vi "Untitled 2.vi"() -> ()   [LabVIEW 2013]
uses:
  <vilib>/Rock Robotics/WPI/Joystick/WPI_JoystickGetSetRefNum.vi
panel:
  in  "Arm Position":enum16{"Arms open", "Arms closed"}(ring)
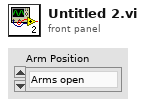
[diagram p1: front panel]
types:
  T1 = typedef "WPI_JoystickDevRef.ctl" = cluster{"Device":T2}
  T2 = typedef "WPI_JoystickDeviceEnum.ctl" = enum16{"USB 1", "USB 2", "USB 3", "USB 4", "Kinect 1", "Kinect 2"}
  T3 = typedef "WPI_JoystickButtonState.ctl" = cluster{"Button 1":bool, "Button 2":bool, "Button 3":bool, "Button 4":bool, "Button 5":bool, "Button 6":bool, "Button 7":bool, "Button 8":bool, "Button 9":bool, "Button 10":bool, "Button 11":bool, "Button 12":bool}
  T4 = typedef "WPI_DigitalInputDevRef.ctl" = cluster{"DevStatus":errorcluster, "DIO Channel":T5, "Digital Module":T6}
  T5 = typedef "FPGA_DIOChannel.ctl" = enum8{"DIO 1", "DIO 2", "DIO 3", "DIO 4", "DIO 5", "DIO 6", "DIO 7", "DIO 8", "DIO 9", "DIO 10", "DIO 11", "DIO 12", "DIO 13", "DIO 14", "Invalid"}
  T6 = typedef "FPGA_TypedefDigitalModule.ctl" = enum16{"Digital Module 1", "Digital Module 2"}
  T7 = typedef "WPI_MotorControlDeviceRef.ctl" = cluster{"DeviceStatus":errorcluster, "Type":enum16{"PWM", "CAN"}, "PWM":cluster{"Digital Module":T6, "PWM Channel":T8, "DeadBand":T9}, "CAN":cluster{"Device Number":u8, "Control Mode":T10, "Semaphore":T11, "Max Vout":dbl}, "Invert":bool, "TransformRef":T12, "InvTransformRef":T12}
  T8 = typedef "FPGA_DIOPWMChannel.ctl" = enum8{"PWM 1", "PWM 2", "PWM 3", "PWM 4", "PWM 5", "PWM 6", "PWM 7", "PWM 8", "PWM 9", "PWM 10", "Invalid"}
  T9 = typedef "WPI_PWMDeadband.ctl" = cluster{"Name":string, "maxPositivePwm":i32, "minPositivePwm":i32, "centerPwm":i32, "maxNegativePwm":i32, "minNegativePwm":i32, "angularRange":u16}
  T10 = typedef "WPI_CANJaguar_ControlMode.ctl" = enum8{"Percent VBus", "Current", "Speed", "Position", "Voltage"}
  T11 = typedef "Semaphore RefNum" = refnum<k1>
  T12 = typedef "WPI_PWMTransform_ConPane.ctl" = refnum<vi>
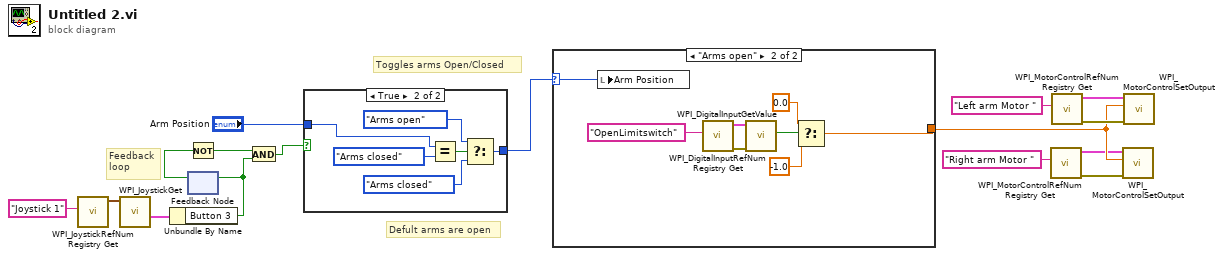
[diagram p0: block diagram]
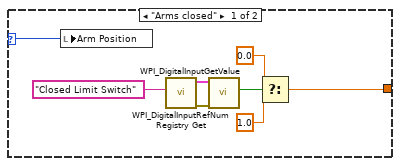
[diagram p3: hidden frame]
diagram:
  # "Toggles arms Open/Closed"
  # "Feedback\nloop"
  # "Defult arms are open"
  n1 = call <vilib>:"WPI_JoystickRefNum Registry Get.vi"("refnum name"="Joystick 1") -> ("JoystickDevRef"=w16:T1)  [unwired: 9 in, 1 out]
  n2 = call <vilib>:"WPI_JoystickGet.vi"("JoystickDevRef"=w16) -> ("Buttons"=w14:T3)  [unwired: 4 in, 2 out]
  n3 = Unbundle By Name(w14) -> ("Button 3"=w3:bool)
  n4 = feedback-in #1(w3) -> ()
  n5 = feedback #1() -> (w5:bool)  [unwired: 1 in]
  n6 = Not(x=w5) -> (.not. x?=w4:bool)
  n7 = And(x=w4, y=w3) -> (x .and. y?=w1:bool)
  n8 = case shown="True" w1 {
    tunnel: [w17 w23] -> w13
    tunnel: "Arm Position" -> [w17 w18]
    frame False {
    }
    frame True {
      n9 = Equal?(x=w18, y=enum16{"Arms open", "Arms closed"}."Arms closed") -> (x = y?=w21:bool)
      n10 = Select(t=enum16{"Arms open", "Arms closed"}."Arms open", s=w21, f=enum16{"Arms open", "Arms closed"}."Arms closed") -> (s? t:f=w23:enum16{"Arms open", "Arms closed"})
    }
  }
  n11 = case shown="\"Arms open\"" w13 {
    selector: w13 -> [w24 w32]
    tunnel: [w25 w33] -> w7
    frame "Arms closed" {
      n12 = local write "Arm Position"(w24) -> ()
      n13 = call <vilib>:"WPI_DigitalInputRefNum Registry Get.vi"("refnum name"="Closed Limit Switch") -> ("error out"=w30:errorcluster, "DigitalInputDevRef"=w31:T4)  [unwired: 9 in]
      n14 = call <vilib>:"WPI_DigitalInputGetValue.vi"("error in (no error)"=w30, "DigitalInputDevRef"=w31) -> ("Value"=w26:bool)  [unwired: 7 in, 2 out]
      n15 = Select(t=0.0, s=w26, f=1.0) -> (s? t:f=w25:dbl)
    }
    frame "Arms open" {
      n16 = local write "Arm Position"(w32) -> ()
      n17 = call <vilib>:"WPI_DigitalInputRefNum Registry Get.vi"("refnum name"="OpenLimitswitch") -> ("error out"=w39:errorcluster, "DigitalInputDevRef"=w38:T4)  [unwired: 9 in]
      n18 = call <vilib>:"WPI_DigitalInputGetValue.vi"("error in (no error)"=w39, "DigitalInputDevRef"=w38) -> ("Value"=w36:bool)  [unwired: 7 in, 2 out]
      n19 = Select(t=0.0, s=w36, f=-1.0) -> (s? t:f=w33:dbl)
    }
  }
  n20 = call <vilib>:"WPI_MotorControlRefNum Registry Get.vi"("refnum name"="Right arm Motor ") -> ("error out"=w8:errorcluster, "MotorControlDevRef"=w6:T7)  [unwired: 9 in]
  n21 = call <vilib>:"WPI_MotorControlRefNum Registry Get.vi"("refnum name"="Left arm Motor ") -> ("error out"=w11:errorcluster, "MotorControlDevRef"=w10:T7)  [unwired: 9 in]
  n22 = call <vilib>:"WPI_MotorControlSetOutput.vi"("error in (no error)"=w8, "Output"=w7, "MotorControlDevRef"=w6) -> ()  [unwired: 6 in, 3 out]
  n23 = call <vilib>:"WPI_MotorControlSetOutput.vi"("error in (no error)"=w11, "Output"=w7, "MotorControlDevRef"=w10) -> ()  [unwired: 6 in, 3 out]
